vi "V-corrected-drive.vi"(8 "R-IN":dbl, 11 "L-IN 2":dbl) -> (0 "Right out":dbl, 3 "Left out":dbl)   [LabVIEW 2015]
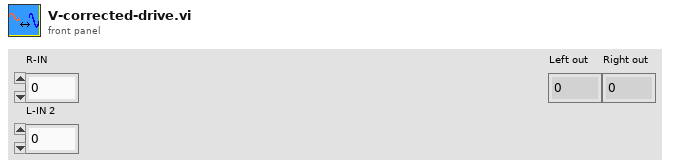
[diagram p1: front panel]
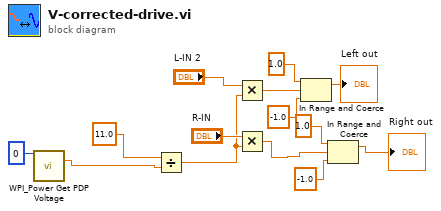
[diagram p0: block diagram]
diagram:
  n1 = call <vilib>:"WPI_Power Get PDP Voltage.vi"("Power Distribution Panel (0)"=u8 0) -> ("voltage (V)"=w4:dbl)  [unwired: 13 in, 1 out]
  n2 = Divide(x=11.0, y=w4) -> (x/y=w8:dbl)
  n3 = Multiply(x="L-IN 2", y=w8) -> (x*y=w14:dbl)
  n4 = Multiply(x="R-IN", y=w8) -> (x*y=w5:dbl)
  n5 = In Range and Coerce(upper limit=1.0, x=w14, lower limit=-1.0) -> (coerced(x)=→"Left out":dbl)  [unwired: 1 out]
  n6 = In Range and Coerce(upper limit=1.0, x=w5, lower limit=-1.0) -> (coerced(x)=→"Right out":dbl)  [unwired: 1 out]
